vi "IsRefnum.vi"(8 "error in":errorcluster, 11 "Defect in":refnum<class "Defect.lvclass">) -> (0 "error out":errorcluster, 2 "IsRefnum":bool, 3 "Defect out":refnum<class "Defect.lvclass">)   [LabVIEW 2021, in "ProligentXMLGenerator.lvlib" / "Defect.lvclass"]
doc: "Returns TRUE if the passed object is valid."
uses:
  Defect.lvclass
  Defect.lvclass/Defect.ctl
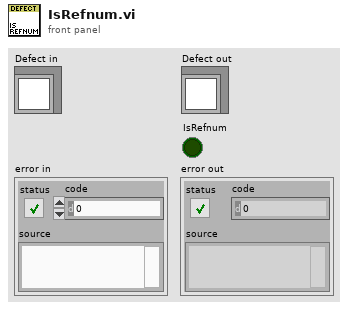
[diagram p1: front panel]
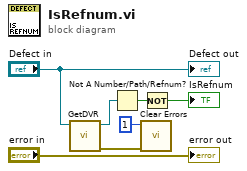
[diagram p0: block diagram]
diagram:
  n1 = call "GetDVR.vi"("Defect"="Defect in") -> ("error out"=w1:errorcluster, "DVRReference"=w3:refnum<data-value>)  [unwired: 9 in]
  n2 = Not A Number/Path/Refnum?(number/path/refnum=w3) -> (NaN/Path/Refnum?=w5:bool)
  n3 = call <vilib>:"Clear Errors.vi"("error in (no error)"=w1, "specific error code to clear (0: all)"=1) -> ()  [unwired: 4 in, 2 out]
  n4 = Not(x=w5) -> (.not. x?=→"IsRefnum":bool)
  "error out" <- "error in"
  "Defect out" <- "Defect in"
